vi "QTI Custom.vi"(9 "num":dbl, 10 "QTI Raw":dbl[](array[numeric])) -> (2 "QTI Binary Custom":bool[](array[boolean]), 5 "size(s)":i32)   [LabVIEW 2020]
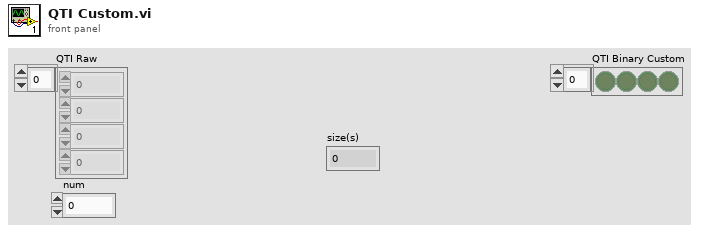
[diagram p1: front panel]
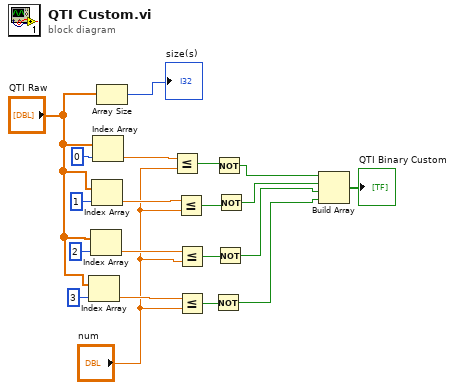
[diagram p0: block diagram]
diagram:
  n1 = Index Array(array="QTI Raw", index=3) -> (element=w11:dbl)
  n2 = Index Array(array="QTI Raw", index=2) -> (element=w12:dbl)
  n3 = Index Array(array="QTI Raw", index=1) -> (element=w13:dbl)
  n4 = Index Array(array="QTI Raw", index=0) -> (element=w14:dbl)
  n5 = Array Size(array="QTI Raw") -> (size(s)=→"size(s)":i32)
  n6 = Less Or Equal?(x=w14, y="num") -> (x <= y?=w5:bool)
  n7 = Less Or Equal?(x=w13, y="num") -> (x <= y?=w8:bool)
  n8 = Less Or Equal?(x=w12, y="num") -> (x <= y?=w7:bool)
  n9 = Less Or Equal?(x=w11, y="num") -> (x <= y?=w6:bool)
  n10 = Not(x=w6) -> (.not. x?=w1:bool)
  n11 = Not(x=w5) -> (.not. x?=w4:bool)
  n12 = Not(x=w7) -> (.not. x?=w2:bool)
  n13 = Not(x=w8) -> (.not. x?=w3:bool)
  n14 = Build Array(w4, w3, w2, w1) -> (→"QTI Binary Custom":bool[])
